vi "getCamRamSegment.vi"(0 "Camera in":refnum<class "Camera.lvclass">, 11 "error in (no error)":errorcluster) -> (4 "Camera out":refnum<class "Camera.lvclass">, 6 "segment":u16, 15 "error out":errorcluster)   [LabVIEW 2019, in "Camera.lvclass"]
doc: "Gets the number of the current RAM segment. Returns an error if camera does not have internal memory."
uses:
  Camera.lvclass
  Camera.lvclass/Camera.ctl
  pco.sdk/StorageControl/StorageControl.lvlib
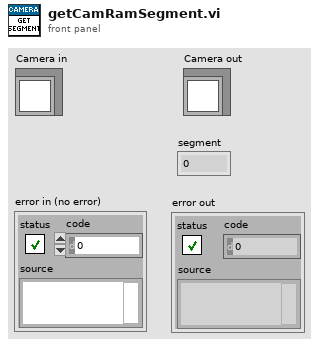
[diagram p1: front panel]
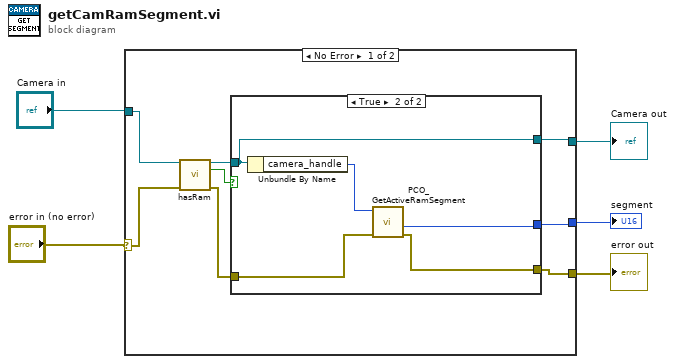
[diagram p0: block diagram]
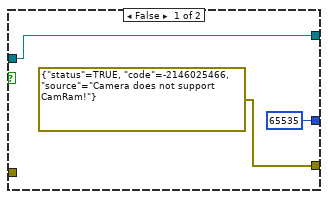
[diagram p2: hidden frame]
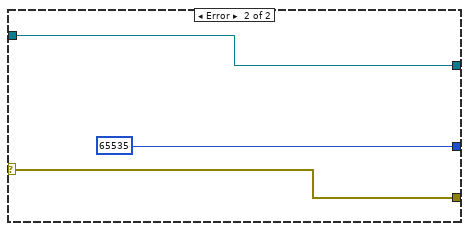
[diagram p3: hidden frame]
diagram:
  n1 = case shown="No Error" "error in (no error)" {
    selector: "error in (no error)" -> [w10 w24]
    tunnel: [w6 w24] -> w3
    tunnel: [w8 w23] -> w4
    tunnel: "Camera in" -> [w9 w23]
    tunnel: [w7 u16 65535 ("dwErr")] -> w1
    frame No Error {
      n2 = call-dynamic "hasRam.vi"("Camera in"=w9, "error in (no error)"=w10) -> ("Camera out"=w13:refnum<class "Camera.lvclass">, "hasRam"=w12:bool, "error out"=w11:errorcluster)  [unwired: 11 in]
      n3 = case shown="True" w12 {
        tunnel: w11 -> [_ w21]
        tunnel: w13 -> [w15 w18]
        tunnel: [errorcluster {"status"=TRUE, "code"=-2146025466, "source"="Camera does not support CamRam!"} ("error constant") w20] -> w6
        tunnel: [w15 w18] -> w8
        tunnel: [u16 65535 ("wActSeg") w17] -> w7
        frame False {
        }
        frame True {
          n4 = Unbundle By Name(w18) -> ("camera_handle"=w19:u64)
          n5 = call "PCO_GetActiveRamSegment.vi"("error in (no error)"=w21, "ph"=w19) -> ("error out"=w20:errorcluster, "wActSeg"=w17:u16)  [unwired: 6 in, 2 out]
        }
      }
    }
    frame Error {
    }
  }
  "error out" <- w3
  "Camera out" <- w4
  "segment" <- w1
